vi "Tearing Down.vi"(7 "Actor in":refnum<class "Actor.lvclass">, 8 "Error in":errorcluster) -> (5 "Actor out":refnum<class "Actor.lvclass">)   [LabVIEW 2020, in "jettl.lvlib"]
uses:
  jettl.lvlib
  Actor/Actor.lvclass
  Transport/Transport.lvclass
  Stopped jettl Msg/Stopped/Stopped.lvlib
  Lifetime.ctl
  Read Self Attributes/Read Self Attributes.lvlib
  Teardown Location.ctl
  Read Self Attributes/Transport.vi
  Stopped jettl Msg/Stopped/Tell Parent.vi
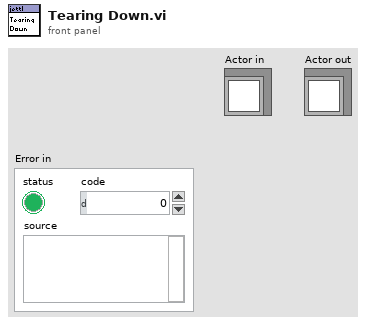
[diagram p1: front panel]
types:
  T1 = typedef "jettl.lvlib/Lifetime.ctl" = enum16{"Init", "Spawn", "Setup", "Teardown Before Running", "Running", "Stop Called", "Stopping With Children", "Stopping Without Children", "Teardown After Running", "Stopped"}
  T2 = typedef "jettl.lvlib/Teardown Location.ctl" = enum16{"Before Running", "After Running"}
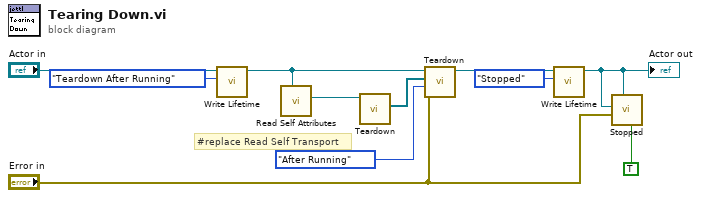
[diagram p0: block diagram]
diagram:
  # "#replace Read Self Transport"
  n1 = call-dynamic "Write Lifetime.vi"("Lifetime"=Lifetime."Teardown After Running", "Actor in"="Actor in") -> ("Actor out"=w6:refnum<class "Actor.lvclass">)  [unwired: 9 in]
  n2 = call-poly "Read Self Attributes.vi"("Actor in"=w6) -> ("Transport"=w5:refnum<class "Transport.lvclass">)  [unwired: 10 in]
  n3 = call-dynamic "Teardown.vi"("Transport in"=w5) -> ("Unheard Msgs"=w11:refnum<class "Msg.lvclass">[])  [unwired: 10 in]
  n4 = call-dynamic "Teardown.vi"("Error in"="Error in", "Teardown Location"=Teardown_Location."After Running", "Unheard Msgs"=w11, "Actor in"=w6) -> ("Actor out"=w2:refnum<class "Actor.lvclass">)  [unwired: 7 in]
  n5 = call-dynamic "Write Lifetime.vi"("Lifetime"=Lifetime."Stopped", "Actor in"=w2) -> ("Actor out"=w8:refnum<class "Actor.lvclass">)  [unwired: 9 in]
  "Actor out" <- w8
  n6 = call-poly "Stopped.vi"("Priority"=TRUE, "Actor in"=w8, "Error"="Error in", "Unified Actor"=w8) -> ()  [unwired: 6 in, 2 out]
